vi "Tracking start report.vi"(3 "Write record when no fit?":refnum<vi>, 4 "Filename":string, 5 "date/time string":string, 6 "Fit type":string, 7 "Move AOIs?":refnum<vi>, 8 "Parameters":T1=[{"Name"="bk", "Specify IV?"=FALSE, "Initial Val."=1.0, "Lower lim."=65000.0, "Upper lim."=0.0, "Fit?"=FALSE}, {"Name"="ht", "Specify IV?"=FALSE, "Initial Val."=0.0, "Lower lim."=65000.0, "Upper lim."=0.0, "Fit?"=FALSE}, {"Name"="xc", "Specify IV?"=FALSE, "Initial Val."=0.0, "Lower lim."=20.0, "Upper lim."=0.0, "Fit?"=FALSE}, {"Name"="yc", "Specify IV?"=FALSE, "Initial Val."=0.0, "Lower lim."=20.0, "Upper lim."=0.0, "Fit?"=FALSE}, {"Name"="wi", "Specify IV?"=FALSE, "Initial Val."=0.0, "Lower lim."=30.0, "Upper lim."=0.0, "Fit?"=FALSE}] {"Upper lim." format="%.2f"; "Lower lim." format="%.2f"; "Initial Val." format="%.2f"}) -> (0 "error out (no error)":errorcluster, 2 "report out":T2)   [LabVIEW 2016]
uses:
  <vilib>/Utility/NIReport.llb/Generate Report Object Reference.ctl
  <vilib>/Utility/NIReport.llb/NI_report.lvclass
  Parameter array.ctt
  <vilib>/Utility/NIReport.llb/HTML Report Image Alignment.ctl
  <vilib>/Utility/NIReport.llb/HTML Report Text Alignment.ctl
  <vilib>/Utility/NIReport.llb/Append Report Text (str wrap).vi
  GLIMPSE Globals.vi
  <vilib>/Utility/NIReport.llb/Append Numeric Table to Report (wrap).vi
  AOI/AOI List Globals.vi
  <vilib>/Utility/NIReport.llb/NI_ReportGenerationCore.lvlib
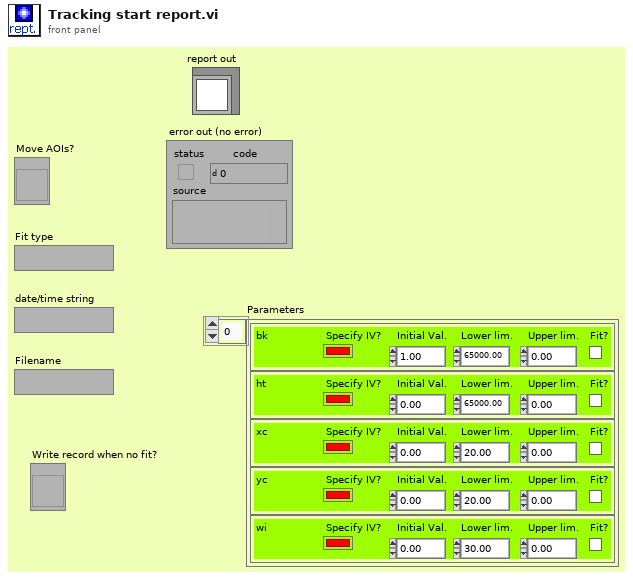
[diagram p1: front panel]
types:
  T1 = typedef "Parameter array.ctt" = cluster{"Name":string, "Specify IV?":bool, "Initial Val.":dbl, "Lower lim.":dbl, "Upper lim.":dbl, "Fit?":bool}[]
  T2 = typedef "Generate Report Object Reference.ctl" = refnum<class "NI_report.lvclass">
  T3 = typedef "NI_ReportGenerationCore.lvlib/HTML Report Text Alignment.ctl" = enum16{"(default)", "LEFT", "CENTER", "RIGHT"}
  T4 = typedef "NI_ReportGenerationCore.lvlib/HTML Report Image Alignment.ctl" = enum16{"(default)", "LEFT", "RIGHT", "TOP", "TEXTTOP", "MIDDLE", "ABSMIDDLE", "BASELINE", "BOTTOM", "ABSBOTTOM"}
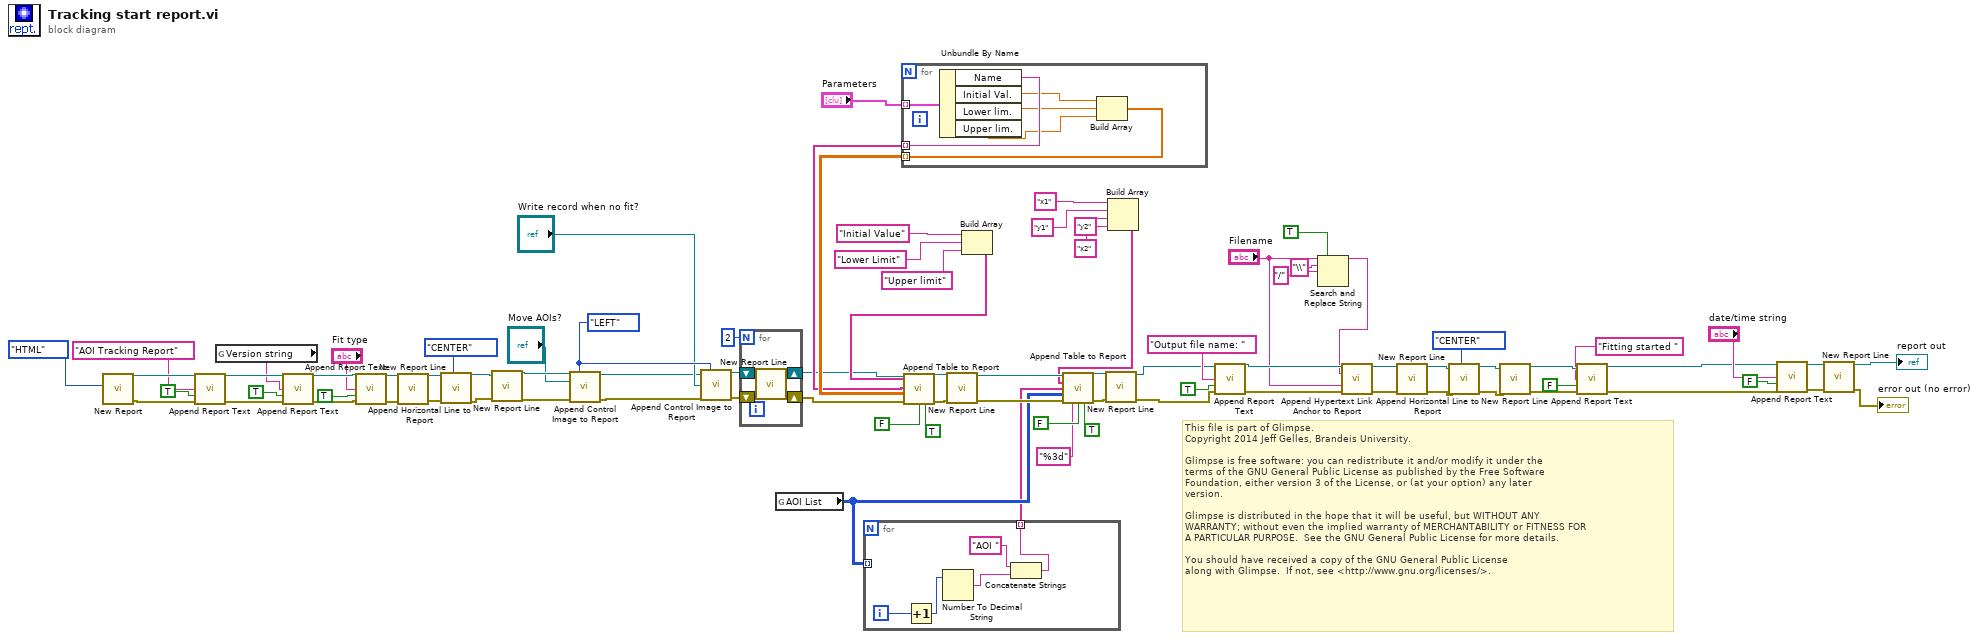
[diagram p0: block diagram]
diagram:
  w23 = HTML_Report_Image_Alignment."LEFT" ("alignment (default)")
  # "This file is part of Glimpse. \nCopyright 2014 Jeff Gelles, Brandeis University.    \n\nGlimpse is free software: you can redistribute it and/or modify it under the \nterms of the GNU General Public License as published by the Free Software \nFoundation, either version 3 of the License, or (at your option) any later \nversion.\n\nGlimpse is distributed in the hope that it will be useful, but WITHOUT ANY \nWARRANTY; without even the implied warranty of MERCHANTABILITY or FITNESS FOR \nA PARTICULAR PURPOSE.  See the GNU General Public License for more details.\n\nYou should have received a copy of the GNU General Public License\nalong with Glimpse.  If not, see <http://www.gnu.org/licenses/>."
  n1 = call <vilib>:"New Report.vi"("report type"=enum16{"Standard Report", "HTML"}."HTML") -> ("report out"=w53:refnum<class "NI_report.lvclass">, "error out"=w54:errorcluster)  [unwired: 5 in, 8 out]
  n2 = call-poly <vilib>:"Append Report Text.vi"("report in"=w53, "text"="AOI Tracking Report", "append on new line? (F)"=TRUE, "error in (no error)"=w54) -> ("report out"=w55:refnum<class "NI_report.lvclass">, "error out"=w56:errorcluster)  [unwired: 2 in, 8 out]
  n3 = global read "GLIMPSE Globals.vi" "Version string"() -> (w48:string)
  n4 = call-poly <vilib>:"Append Report Text.vi"("report in"=w55, "text"=w48, "append on new line? (F)"=TRUE, "error in (no error)"=w56) -> ("report out"=w73:refnum<class "NI_report.lvclass">, "error out"=w75:errorcluster)  [unwired: 2 in, 8 out]
  n5 = call-poly <vilib>:"Append Report Text.vi"("report in"=w73, "text"="Fit type", "append on new line? (F)"=TRUE, "error in (no error)"=w75) -> ("report out"=w74:refnum<class "NI_report.lvclass">, "error out"=w76:errorcluster)  [unwired: 2 in, 8 out]
  n6 = call-dynamic "New Report Line.vi"("report in"=w74, "error in (no error)"=w76) -> ("report out"=w61:refnum<class "NI_report.lvclass">, "error out"=w64:errorcluster)  [unwired: 1 in, 11 out]
  n7 = call-dynamic "Append Horizontal Line to Report.vi"("report in"=w61, "align (default)"=HTML_Report_Text_Alignment."CENTER", "error in (no error)"=w64) -> ("report out"=w62:refnum<class "NI_report.lvclass">, "error out"=w63:errorcluster)  [unwired: 5 in, 6 out]
  n8 = call-dynamic "New Report Line.vi"("report in"=w62, "error in (no error)"=w63) -> ("report out"=w87:refnum<class "NI_report.lvclass">, "error out"=w86:errorcluster)  [unwired: 1 in, 11 out]
  n9 = call-dynamic "Append Control Image to Report.vi"("report in"=w87, "alignment (default)"=w23, "ctrl reference"="Move AOIs?", "error in (no error)"=w86) -> ("report out"=w3:refnum<class "NI_report.lvclass">, "error out"=w2:errorcluster)  [unwired: 4 in, 6 out]
  n10 = call-dynamic "Append Control Image to Report.vi"("report in"=w3, "alignment (default)"=w23, "ctrl reference"="Write record when no fit?", "error in (no error)"=w2) -> ("report out"=w24:refnum<class "NI_report.lvclass">, "error out"=w25:errorcluster)  [unwired: 4 in, 6 out]
  n11 = for {
    N: 2 -> [_]
    shift-right: [w89] -> w21
    shift-left: w24 -> [w90]
    shift-right: [w88] -> w20
    shift-left: w25 -> [w91]
    n12 = call-dynamic "New Report Line.vi"("report in"=w90, "error in (no error)"=w91) -> ("report out"=w89:refnum<class "NI_report.lvclass">, "error out"=w88:errorcluster)  [unwired: 1 in, 11 out]
  }
  n13 = global read "AOI List Globals.vi" "AOI List"() -> (w5:u16[][])
  n14 = for {
    tunnel: w5 -> [_] mode=indexing
    tunnel: [w93] -> w4 mode=indexing
    i -> [w96]
    n15 = Increment(x=w96) -> (x+1=w92:i32)
    n16 = Number To Decimal String(number=w92) -> (decimal integer string=w94:string)  [unwired: 1 out]
    n17 = Concatenate Strings("AOI " ("string"), w94) -> (w93:string)
  }
  n18 = for {
    tunnel: "Parameters" -> [w102] mode=indexing
    tunnel: [w101] -> w77 mode=indexing
    tunnel: [w97] -> w78 mode=indexing
    n19 = Unbundle By Name(w102) -> ("Name"=w101:string, "Initial Val."=w100:dbl, "Lower lim."=w99:dbl, "Upper lim."=w98:dbl)
    n20 = Build Array(w100, w99, w98) -> (w97:dbl[])
  }
  n21 = Build Array("Initial Value" ("string"), "Lower Limit" ("string"), "Upper limit" ("string")) -> (w82:string[])
  n22 = call-poly <vilib>:"Append Table to Report.vi"("report in"=w21, "column headers"=w82, "row headers"=w77, "numerical data"=w78, "error in (no error)"=w20, "separate page?"=FALSE, "show grid lines"=TRUE) -> ("report out"=w50:refnum<class "NI_report.lvclass">, "error out"=w49:errorcluster)  [unwired: 3 in, 4 out]
  n23 = call-dynamic "New Report Line.vi"("report in"=w50, "error in (no error)"=w49) -> ("report out"=w13:refnum<class "NI_report.lvclass">, "error out"=w15:errorcluster)  [unwired: 1 in, 11 out]
  n24 = Build Array("x1" ("string"), "y1" ("string"), "x2" ("string"), "y2" ("element")) -> (w6:string[])
  n25 = call-poly <vilib>:"Append Table to Report.vi"("report in"=w13, "column headers"=w6, "row headers"=w4, "numerical data"=w5, "error in (no error)"=w15, "format string (%.3f)"="%3d" ("format string (%.2f)"), "separate page?"=FALSE, "show grid lines"=TRUE) -> ("report out"=w17:refnum<class "NI_report.lvclass">, "error out"=w16:errorcluster)  [unwired: 2 in, 4 out]
  n26 = call-dynamic "New Report Line.vi"("report in"=w17, "error in (no error)"=w16) -> ("report out"=w12:refnum<class "NI_report.lvclass">, "error out"=w14:errorcluster)  [unwired: 1 in, 11 out]
  n27 = call-poly <vilib>:"Append Report Text.vi"("report in"=w12, "text"="Output file name: ", "append on new line? (F)"=TRUE, "error in (no error)"=w14) -> ("report out"=w32:refnum<class "NI_report.lvclass">, "error out"=w33:errorcluster)  [unwired: 2 in, 8 out]
  n28 = Search and Replace String(replace all?=TRUE ("replace all? (F)"), input string="Filename", search string="\\", replace string="/" ("replace string (\"\")")) -> (result string=w26:string)  [unwired: 1 in, 6 out]
  n29 = call-dynamic "Append Hypertext Link Anchor to Report.vi"("report in"=w32, "URL of link - href"=w26, "link text"="Filename", "error in (no error)"=w33) -> ("report out"=w31:refnum<class "NI_report.lvclass">, "error out"=w34:errorcluster)  [unwired: 1 in, 9 out]
  n30 = call-dynamic "New Report Line.vi"("report in"=w31, "error in (no error)"=w34) -> ("report out"=w65:refnum<class "NI_report.lvclass">, "error out"=w68:errorcluster)  [unwired: 1 in, 11 out]
  n31 = call-dynamic "Append Horizontal Line to Report.vi"("report in"=w65, "align (default)"=HTML_Report_Text_Alignment."CENTER", "error in (no error)"=w68) -> ("report out"=w66:refnum<class "NI_report.lvclass">, "error out"=w69:errorcluster)  [unwired: 5 in, 6 out]
  n32 = call-dynamic "New Report Line.vi"("report in"=w66, "error in (no error)"=w69) -> ("report out"=w67:refnum<class "NI_report.lvclass">, "error out"=w70:errorcluster)  [unwired: 1 in, 11 out]
  n33 = call-poly <vilib>:"Append Report Text.vi"("report in"=w67, "text"="Fitting started ", "append on new line? (F)"=FALSE, "error in (no error)"=w70) -> ("report out"=w43:refnum<class "NI_report.lvclass">, "error out"=w44:errorcluster)  [unwired: 2 in, 8 out]
  n34 = call-poly <vilib>:"Append Report Text.vi"("report in"=w43, "text"="date/time string", "append on new line? (F)"=FALSE, "error in (no error)"=w44) -> ("report out"=w42:refnum<class "NI_report.lvclass">, "error out"=w41:errorcluster)  [unwired: 2 in, 8 out]
  n35 = call-dynamic "New Report Line.vi"("report in"=w42, "error in (no error)"=w41) -> ("report out"=→"report out":refnum<class "NI_report.lvclass">, "error out"=→"error out (no error)":errorcluster)  [unwired: 1 in, 11 out]
